vi "Pulse Demo.vi"() -> ()   [LabVIEW 2023]
doc: "Simulates a transmission and receiver system. The example simulates the transmission of a pulse in a noisy environment based upon basic communication theory, with x(t) representing the pulse in question.\n\nThe Transmitter generates the signal x(t) and modulates it to create a signal of the form:\nx[m](t) = x(t)cos(2(pi)f[c]t)\nwhere f[c] is the carrier frequency.\n\nThe Noise, whose icon is a lightning bolt hitting the wire, then corrupts the transmitted signal with a noise signal. The Noise signal is:\nx[n](t) = x[m](t) + n(t) = x(t)cos(2(pi)f[c]t) + n(t)\nwhere n(t) is an uncorrelated noise signal.\n\nThe Receiver, whose icon is a parabolic antenna, receives and demodulates the noisy pulse. Because the carrier frequency is known, you can demodulate the signal through a heterodyning procedure. Expanding the following terms:\ny(t) = 2x[n](t)cos(2(pi)f[c]t) + n(t)\n = 2 [x(t)cos(2(pi)f[c]t) + n(t)] cos(2(pi)f[c]t)\n = 2x(t)cos^2(2(pi)f[c]t) + n(t)cos(2(pi)f[c]t)\n = x(t) + x(t)cos(4(pi)f[c]t) + 2n(t)cos(2(pi)f[c]t)\n\nThe signal y(t) contains the original signal x(t), which contains the pulse information plus two modulated signals in the upper portion of the spectrum, one at fc and the other one at 2fc. To extract x(t) from y(t), you can use a low pass filter with a cutoff frequency less than the carrier frequency:\nx(t) = approximately Lowpass[y(t)]"
uses:
  <vilib>/Analysis/3filter.llb/Bessel Filter (DBL).vi
  <vilib>/Analysis/NI_AALBase.lvlib
panel:
  in  "Tab Control":T1(tab)
  out "Input Signal":dbl[](graph)
  out "Modulated Signal":dbl[](graph)
  in  "Pulse Delay":i32(knob)=64 scale=0.0..200.0
  in  "Duration":i32(slide)=128 scale=0.0..200.0
  in  "cycles per samples":i32(slide)=4 scale=4.0..10.0
  in  "Additive Noise":dbl(knob)=0.22867271200946546 scale=0.0..1.0 scale format="%0.1f"
  out "Distorted Modulated Signal":dbl[](graph)
  out "Demodulated Signal":i16[](graph)
  out "Demodulated and filtered Signal":dbl[][](graph)
  in  "low cutoff freq: fl":dbl=0.125 format="%0.4f"
  in  "Filter Order":i32(slide)=5 scale=1.0..20.0
  in  "Threshold to detect signal":dbl=0.5
  in  "Stop":bool
  # "Overview: Simulates transmission of a pulse in a noisy environment based upon basic communication theory.\nRequirements: LabVIEW Full Development System\nInstructions: \n1. Run the VI and navigate the tabs to observe the different steps in the generation, transmission, and reception of the pulse.\n2. Change parameters and verify how it modifies the resulting signals.\n3. Click Stop to stop the VI."
  # "Signal Generation"
  # "Modulation"
  # "Signal Corruption (noise)"
  # "Transmission noise"
  # "Reception"
  # "Low-Pass Filter"
  # "After threshold Function"
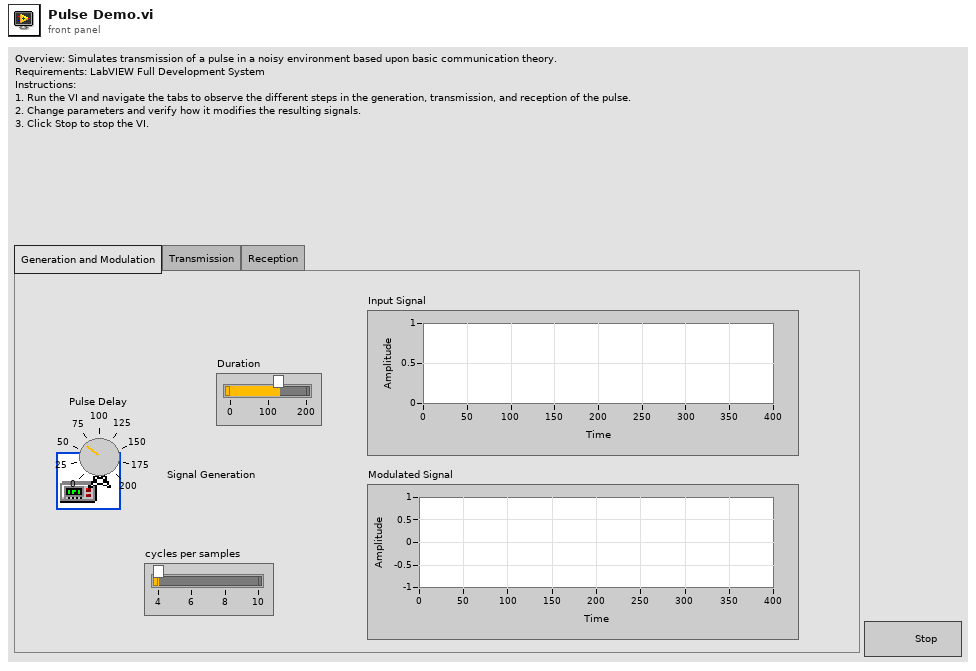
[diagram p1: front panel]
types:
  T1 = enum32{"Generation and Modulation", "Transmission", "Reception"}
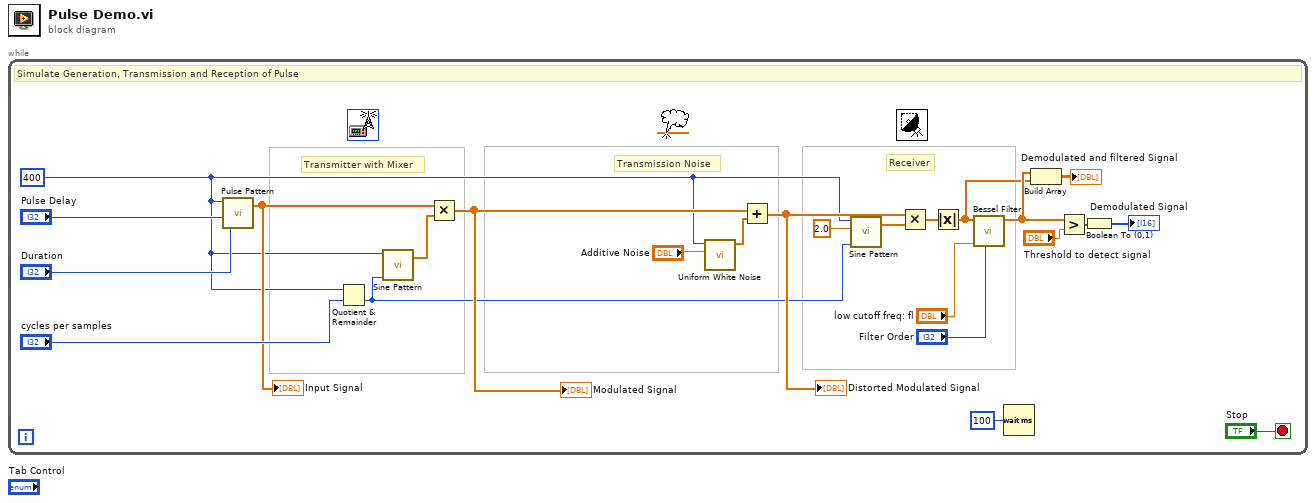
[diagram p0: block diagram]
diagram:
  n1 = while {
    stop <- "Stop" stop-if-true
    w8 = 400 ("Samples")
    # "Receiver"
    # "Transmitter with Mixer"
    # "Transmission Noise"
    # "Simulate Generation, Transmission and Reception of Pulse"
    n2 = call <vilib>:"Pulse Pattern.vi"("width"="Duration", "delay"="Pulse Delay", "samples"=w8) -> ("Pulse Pattern"=w19:dbl[])  [unwired: 1 in, 1 out]
    "Input Signal" <- w19
    n3 = Quotient & Remainder(x=w8, y="cycles per samples") -> (floor(x/y)=w9:i32)  [unwired: 1 out]
    n4 = call <vilib>:"Sine Pattern.vi"("cycles"=w9, "samples"=w8) -> ("Sinusoidal Pattern"=w23:dbl[])  [unwired: 2 in, 1 out]
    n5 = Multiply(x=w19, y=w23) -> (x*y=w13:dbl[])
    "Modulated Signal" <- w13
    n6 = call <vilib>:"Uniform White Noise.vi"("amplitude"="Additive Noise", "samples"=w8) -> ("uniform white noise"=w18:dbl[])  [unwired: 8 in, 1 out]
    n7 = Add(x=w13, y=w18) -> (x+y=w12:dbl[])
    "Distorted Modulated Signal" <- w12
    n8 = call <vilib>:"Sine Pattern.vi"("cycles"=w9, "amplitude"=2.0, "samples"=w8) -> ("Sinusoidal Pattern"=w15:dbl[])  [unwired: 1 in, 1 out]
    n9 = Multiply(x=w12, y=w15) -> (x*y=w16:dbl[])
    n10 = Absolute Value(x=w16) -> (abs(x)=w1:dbl[])
    n11 = call-poly <vilib>:"Bessel Filter.vi"("order"="Filter Order", "low cutoff freq: fl"="low cutoff freq: fl", "X"=w1) -> ("Filtered X"=w6:dbl[])  [unwired: 5 in, 1 out]
    n12 = Wait (ms)(milliseconds to wait=u32 100) -> ()  [unwired: 1 out]
    n13 = Build Array(w6, w1) -> (→"Demodulated and filtered Signal":dbl[][])
    n14 = Greater?(x=w6, y="Threshold to detect signal") -> (0:w4:bool[])
    n15 = Boolean To (0,1)(Boolean=w4) -> (0, 1=→"Demodulated Signal":i16[])
  }
